vi "故障码字段定义.vi"(10 "首次调用？":bool, 11 "故障代码":u16(ring) items=["无故障", "电机故障", "温度故障", "通讯故障", "滴定故障"]) -> (3 "data":T1)   [LabVIEW 2016, in "挥发酚.lvlib"]
uses:
  Alarm interface/Alarm interface.lvlib
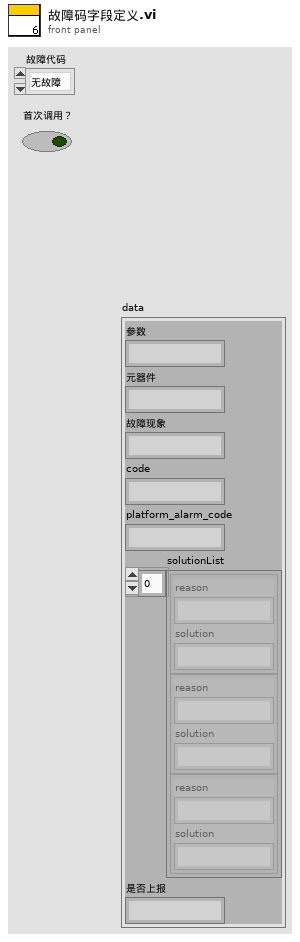
[diagram p1: front panel]
types:
  T1 = typedef "Alarm interface.lvlib/报警短信语音交互.ctl" = cluster{"参数":string, "元器件":string, "故障现象":string, "code":string, "platform_alarm_code":string, "solutionList":cluster{"reason":string, "solution":string}[], "是否上报":string}
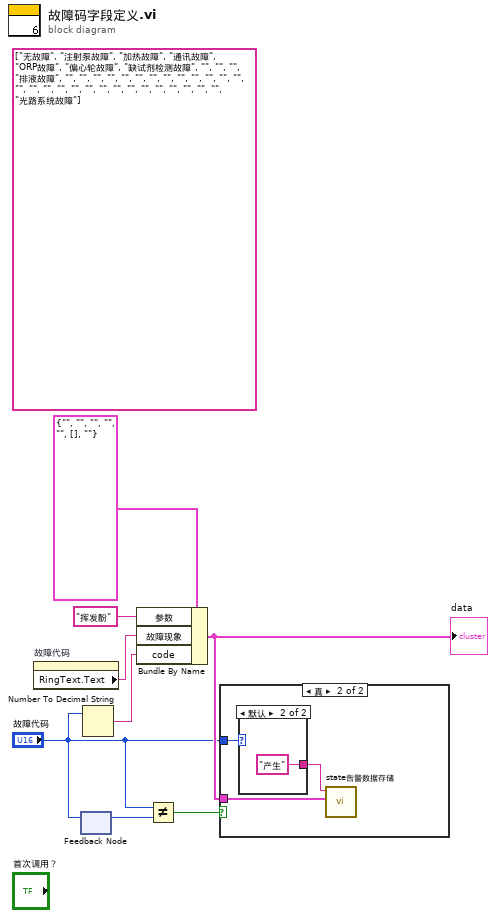
[diagram p0: block diagram]
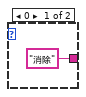
[diagram p3: hidden frame]
diagram:
  (unwired) string[] ["无故障", "注射泵故障", "加热故障", "通讯故障", "ORP故障", "偏心轮故障", "缺试剂检测故障", "", "", "", "排液故障", "", "", "", "", "", "", "", "", "", "", "", "", "", "", "", "", "", "", "", "", "", "", "", "", "", "", "", "", "光路系统故障"]
  n1 = property on="故障代码" class="Ring (严格)"() -> ("RingText.Text"=w7:string)  [unwired: 2 in, 2 out]
  n2 = feedback #1() -> (w4:u16)  [unwired: 1 in]
  n3 = feedback-in #1("故障代码") -> ()
  n4 = Number To Decimal String(number="故障代码") -> (decimal integer string=w6:string)  [unwired: 1 in]
  n5 = Bundle By Name(cluster=T1 {"参数"="", "元器件"="", "故障现象"="", "code"="", "platform_alarm_code"="", "solutionList"=[], "是否上报"=""} ("data"), "参数"="挥发酚", "故障现象"=w7, "code"=w6) -> (w2:T1)
  "data" <- w2
  n6 = Not Equal?(x="故障代码", y=w4) -> (x != y?=w3:bool)
  n7 = case shown="真" w3 {
    tunnel: "故障代码" -> [_ w11]
    tunnel: w2 -> [_ w10]
    frame False {
    }
    frame True {
      n8 = case shown="默认" w11 {
        tunnel: ["消除" "产生"] -> w9
        frame 0 {
        }
        frame Default {
        }
      }
      n9 = call "state告警数据存储.vi"("data"=w10, "state"=w9) -> ()  [unwired: 9 in, 1 out]
    }
  }
